vi "Demo_XControl.vi"() -> ()   [LabVIEW 2013]
uses:
  Bit by Bit Adjust_Xcontrol.xctl
panel:
  out "Output value":dbl format="%#_6f"
  in  "Bit by Bit Adjust_Xcontrol":dbl(xcontrol)
  in  "Stop":bool
  out "Value_Display":i32 format="%05d"
  # "%"
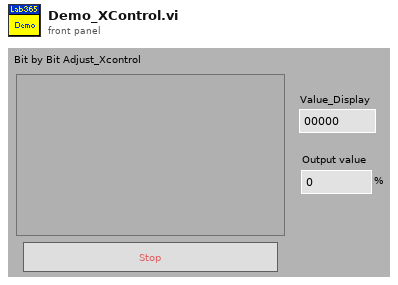
[diagram p1: front panel]
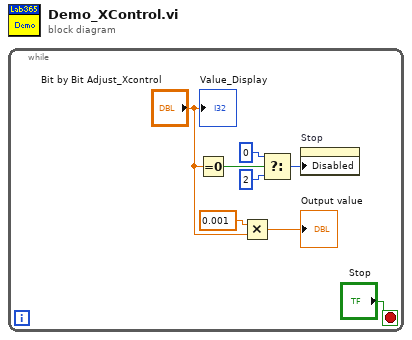
[diagram p0: block diagram]
diagram:
  n1 = while {
    stop <- "Stop" stop-if-true
    n2 = Equal To 0?(x="Bit by Bit Adjust_Xcontrol") -> (x = 0?=w5:bool)
    n3 = Multiply(x=0.001, y="Bit by Bit Adjust_Xcontrol") -> (x*y=→"Output value":dbl)
    n4 = Select(t=i8 0, s=w5, f=i8 2) -> (s? t:f=w4:i8)
    n5 = property on="Stop" class="Bool"("Disabled"=w4) -> ()  [unwired: 2 in, 2 out]
    "Value_Display" <- "Bit by Bit Adjust_Xcontrol"
  }
